vi "triggeredsequencetest.vi"() -> ()   [LabVIEW 2009]
panel:
  out "Trigger number":dbl
  in  "camerasource":string="img0"
  in  "Trigger action":u32(ring)=1 items=["Disabled", "Trigger start of acquisition", "Trigger start of each buffer list", "Trigger each buffer", "Trigger each line (linescan)", "Trigger end of acquisition"]
  in  "Trigger Type":u32(ring) items=["External", "RTSI", "ISO In"]
  in  "Data frames / trigger":dbl=10.0
  in  "Video Frames / Data frame":dbl=15.0
  in  "Manual (up) or automatic (down)":bool
  in  "Or, read path automatically from:":path=path "\\\\Foghorn.bio.brandeis.edu\\remote"
  in  "Manual save directory":string
  in  "Manual save path":path
  in  "stop":bool
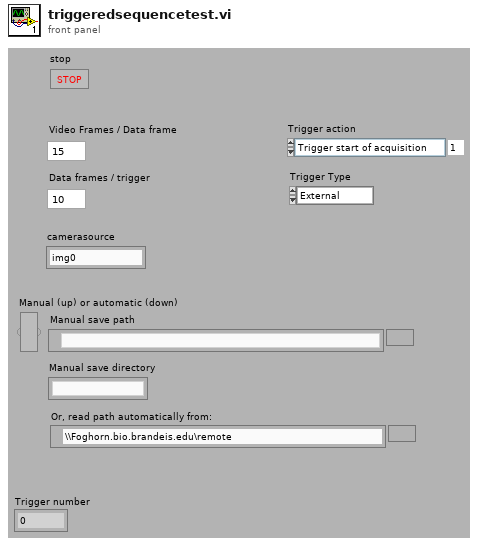
[diagram p1: front panel]
types:
  T1 = typedef "IMAQ Image.ctl" = refnum<image>
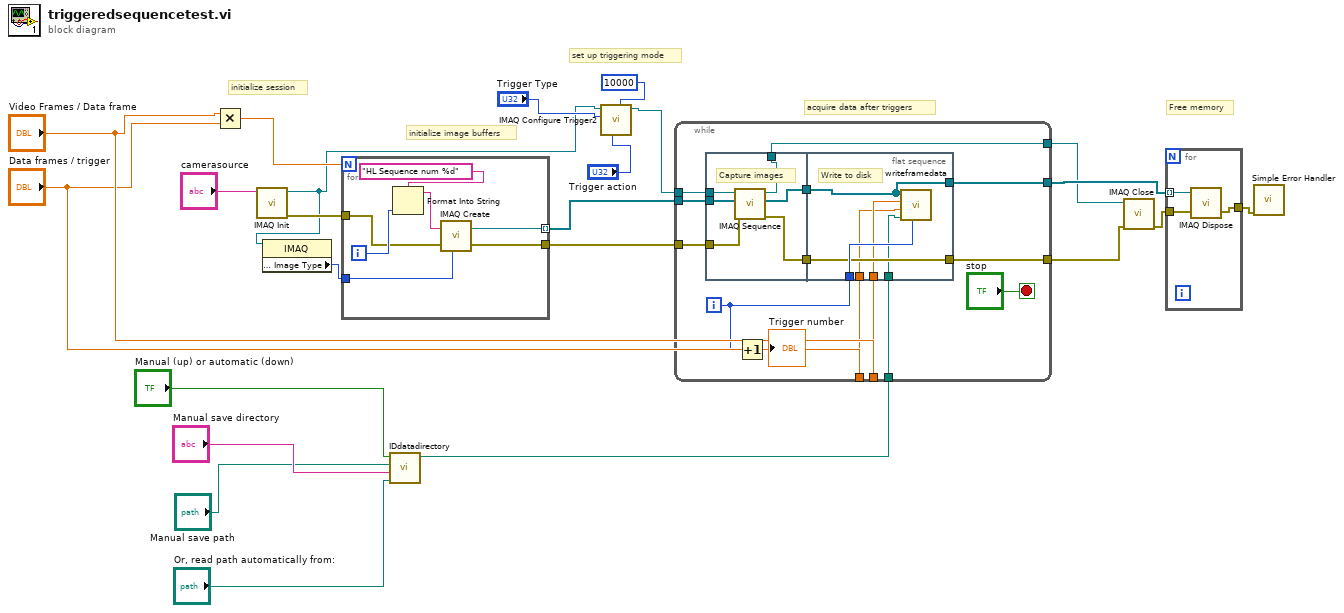
[diagram p0: block diagram]
diagram:
  # "set up triggering mode"
  # "acquire data after triggers"
  # "initialize image buffers"
  # "initialize session"
  # "Free memory"
  n1 = Multiply(x="Video Frames / Data frame", y="Data frames / trigger") -> (x*y=w8:dbl)
  n2 = call <vilib>:"IMAQ Init.vi"("Interface Name"="camerasource") -> ("error out"=w16:errorcluster, "IMAQ Session Out"=w1:refnum<k11>)  [unwired: 9 in]
  n3 = property class="IMAQ"(reference=w1) -> ("Image Parameters : Image Type"=w18:u32)  [unwired: 1 in, 2 out]
  n4 = for {
    N: w8 -> [_]
    tunnel: w18 -> [w27]
    tunnel: [w26] -> w17 mode=indexing
    tunnel: w16 -> [w25]
    tunnel: [w24] -> w15
    i -> [w30]
    n5 = Format Into String(format string="HL Sequence num %d", w30) -> (resulting string=w28:string)  [unwired: 2 in, 1 out]
    n6 = call "IMAQ Create"("Image Name"=w28, "Image Type"=w27, "error in (no error)"=w25) -> ("New Image"=w26:T1, "error out"=w24:errorcluster)  [unwired: 2 in]
  }
  n7 = call "IDdatadirectory.vi"("Read path automatically from:"="Or, read path automatically from:", "Directory"="Manual save directory", "Save path"="Manual save path", "Manual or automatic"="Manual (up) or automatic (down)") -> ("Outputpath"=w9:path)  [unwired: 7 in]
  n8 = call <vilib>:"IMAQ Configure Trigger2.vi"("Frame timeout (ms)"=u32 10000, "Trigger action"="Trigger action", "Trigger Type"="Trigger Type", "IMAQ Session In"=w1) -> ("IMAQ Session Out"=w2:refnum<k11>)  [unwired: 6 in, 1 out]
  n9 = while {
    tunnel: w15 -> [w44]
    tunnel: w2 -> [w43]
    tunnel: w17 -> [w42]
    tunnel: [w39] -> w21
    tunnel: [w38] -> w22
    tunnel: [w36] -> w23
    tunnel: w9 -> [w35]
    tunnel: "Video Frames / Data frame" -> [w34]
    tunnel: "Data frames / trigger" -> [w33]
    i -> [w31]
    stop <- "stop" stop-if-true
    n10 = flat-sequence {
      tunnel: w44 -> [w50]
      tunnel: w43 -> [w49]
      tunnel: w42 -> [w48]
      tunnel: [w47] -> w40
      tunnel: [w46] -> w39
      tunnel: [w45] -> w37
      tunnel: w40 -> [w54]
      tunnel: w31 -> [w56]
      tunnel: [w55] -> w38
      tunnel: w37 -> [w55]
      tunnel: [w54] -> w36
      tunnel: w35 -> [w53]
      tunnel: w34 -> [w52]
      tunnel: w33 -> [w51]
      frame #0 {
        # "Capture images"
        n11 = call <vilib>:"IMAQ Sequence.vi"("error in (no error)"=w50, "Images In"=w48, "IMAQ Session In"=w49) -> ("error out"=w45:errorcluster, "Images Out"=w47:T1[], "IMAQ Session Out"=w46:refnum<k11>)  [unwired: 6 in]
      }
      frame #1 {
        # "Write to disk"
        n12 = call "writeframedata.vi"("trigger number"=w56, "pathname"=w53, "data frames / trigger"=w51, "video frames / data frame"=w52, "Images In"=w54) -> ()  [unwired: 7 in]
      }
    }
    n13 = Increment(x=w31) -> (x+1=→"Trigger number":i32)
  }
  n14 = call <vilib>:"IMAQ Close.vi"("error in (no error)"=w22, "IMAQ Session In"=w21) -> ("error out"=w20:errorcluster)  [unwired: 9 in]
  n15 = for {
    tunnel: w23 -> [w59] mode=indexing
    tunnel: w20 -> [w58]
    tunnel: [w57] -> w19
    n16 = call "IMAQ Dispose"("Image"=w59, "error in (no error)"=w58) -> ("error out"=w57:errorcluster)  [unwired: 4 in]
  }
  n17 = call <vilib>:"Simple Error Handler.vi"("error in (no error)"=w19) -> ()  [unwired: 4 in, 5 out]
